vi "IHL_Inspecting Helper.vi"(8 "error in (no error)":errorcluster, 10 "Inspect Helper Loop Data":T2={"IHL State"=enum."Init", "Timeout"=0, "Loop Count"=0, "Start Sample No."=0, "No. Samples"=0, "Collecting Data"=FALSE, "Success Flag"=FALSE, "Inspect Status "={"Ready"=FALSE, "Inspecting"=FALSE, "Cancel"=FALSE}, "Status"=0, "Encoder Count"=0, "PosToStartScan"=50800, "ScanLength"=50800, "MaxSamples"=50800, "PosToEndScan"=0, "data value reference"=refnum, "Block Cnt notifier out"=refnum, "EventLog"=refnum}) -> (0 "error out":errorcluster, 2 "Inspect Helper Loop Data out":T2={"IHL State"=enum."Init", "Timeout"=0, "Loop Count"=0, "Start Sample No."=0, "No. Samples"=0, "Collecting Data"=FALSE, "Success Flag"=FALSE, "Inspect Status "={"Ready"=FALSE, "Inspecting"=FALSE, "Cancel"=FALSE}, "Status"=0, "Encoder Count"=0, "PosToStartScan"=50800, "ScanLength"=50800, "MaxSamples"=50800, "PosToEndScan"=0, "data value reference"=refnum, "Block Cnt notifier out"=refnum, "EventLog"=refnum}, 3 "State String":string="IHL:Timeout: Inspecting")   [LabVIEW 2015, in "Tool Module.lvlib"]
uses:
  Tool Module.lvlib
  _IHL Data Cluster--typedef.ctl
  Event Logger Library/Event Log/EventLog.lvclass
  _IHL SM Enum--typedef.ctl
  _IHL Status Update Cluster--typedef.ctl
  _Sample Data Rtn Cluster--typedef.ctl
  _Inspection Limits cluster--typedef.ctl
panel:
  out "latest notification":T1
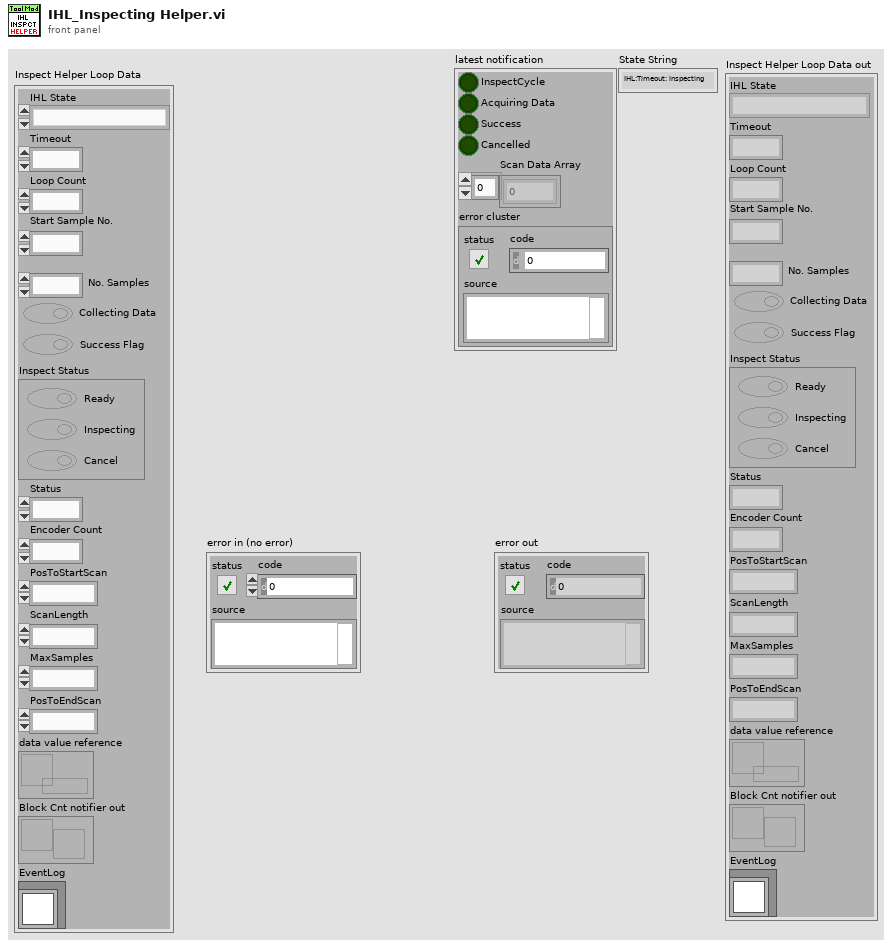
[diagram p1: front panel]
types:
  T1 = typedef "Tool Module.lvlib/_Sample Data Rtn Cluster--typedef.ctl" = cluster{"InspectCycle":bool, "Acquiring Data":bool, "Success":bool, "Cancelled":bool, "Scan Data Array":u32[], "error cluster":errorcluster}
  T2 = typedef "Tool Module.lvlib/_IHL Data Cluster--typedef.ctl" = cluster{"IHL State":T3, "Timeout":i32, "Loop Count":i32, "Start Sample No.":u32, "No. Samples":i32, "Collecting Data":bool, "Success Flag":bool, "Inspect Status ":T4, "Status":u16, "Encoder Count":i32, "PosToStartScan":i32, "ScanLength":i32, "MaxSamples":i32, "PosToEndScan":i32, "data value reference":refnum<data-value>, "Block Cnt notifier out":refnum<notifier>, "EventLog":refnum<class "EventLog.lvclass">}
  T3 = typedef "Tool Module.lvlib/_IHL SM Enum--typedef.ctl" = enum16{"Init", "Set Motion Speed", "Move To Scan Start", "Wait for Motion Out", "Wait for Start Pos", "Inspect: START", "Wait for Motion IN", "Wait for Inspect Range", "Inspecting", "Inspect: STOP"}
  T4 = typedef "Tool Module.lvlib/_IHL Status Update Cluster--typedef.ctl" = cluster{"Ready":bool, "Inspecting":bool, "Cancel":bool}
  T5 = typedef "Tool Module.lvlib/_Inspection Limits cluster--typedef.ctl" = cluster{"MaxSamples":i32, "PosToStartScan":i32, "PosToEndScan":i32, "ScanLength":i32}
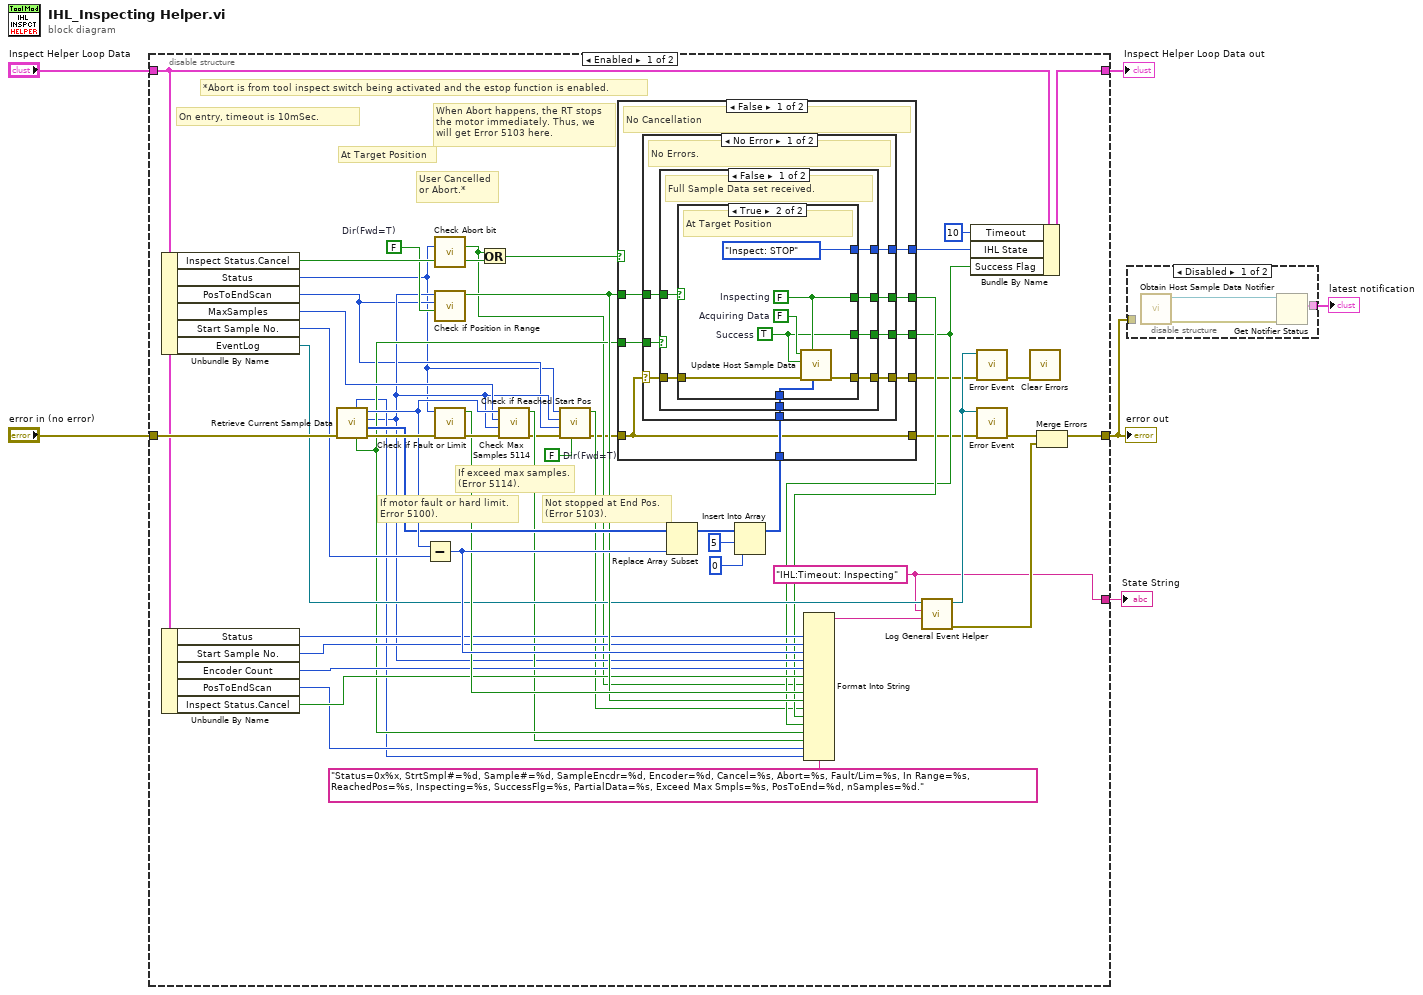
[diagram p0: block diagram]
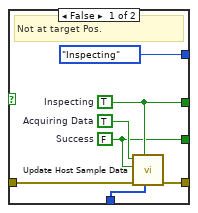
[diagram p3: hidden frame]
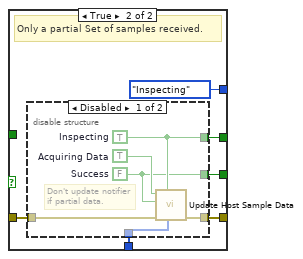
[diagram p4: hidden frame]
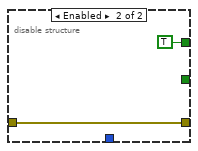
[diagram p5: hidden frame]
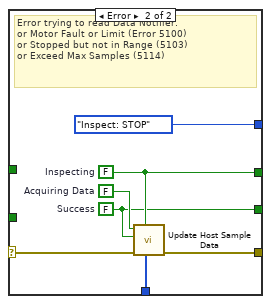
[diagram p6: hidden frame]
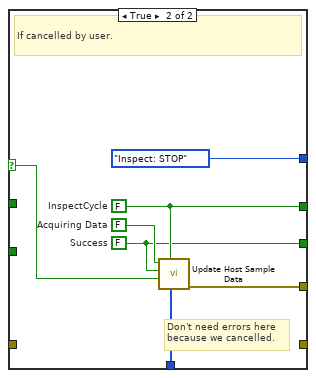
[diagram p7: hidden frame]
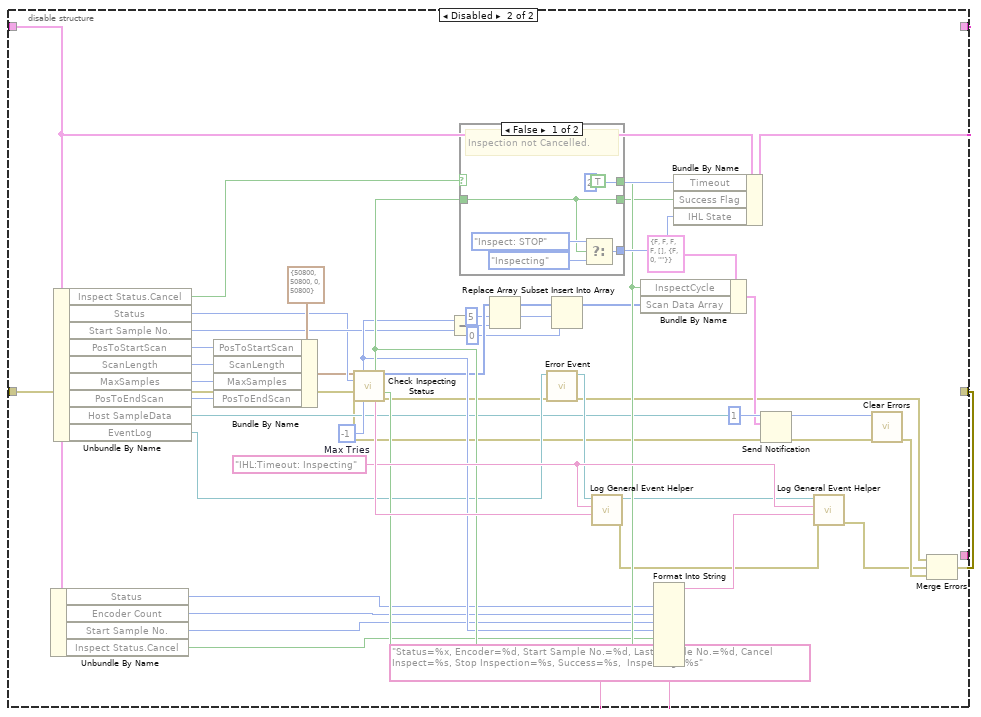
[diagram p8: hidden frame]
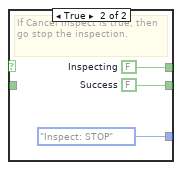
[diagram p9: hidden frame]
diagram:
  n1 = disable-structure shown="Enabled" {
    disable-tunnel: "Inspect Helper Loop Data" -> [w29 w125]
    disable-tunnel: [w30 w124] -> w5
    disable-tunnel: [w28 w123] -> w1
    disable-tunnel: "error in (no error)" -> [w55 w122]
    disable-tunnel: [w9 _] -> w2
    frame Enabled {
      w22 = FALSE  # Dir(Fwd=T)
      w9 = "IHL:Timeout: Inspecting"
      w53 = FALSE  # Dir(Fwd=T)
      # "When Abort happens, the RT stops the motor immediately. Thus, we will get Error 5103 here."
      # "On entry, timeout is 10mSec."
      # "Not stopped at End Pos.\n(Error 5103)."
      # "*Abort is from tool inspect switch being activated and the estop function is enabled."
      # "User Cancelled\nor Abort.*"
      # "At Target Position"
      # "If motor fault or hard limit.\nError 5100)."
      # "If exceed max samples.\n(Error 5114)."
      n2 = Unbundle By Name(w29) -> ("Inspect Status.Cancel"=w56:bool, "Status"=w19:u16, "PosToEndScan"=w20:i32, "MaxSamples"=w34:i32, "Start Sample No."=w41:u32, "EventLog"=w33:refnum<class "EventLog.lvclass">)
      n3 = Unbundle By Name(w29) -> ("Status"=w37:u16, "Start Sample No."=w36:u32, "Encoder Count"=w35:i32, "PosToEndScan"=w25:i32, "Inspect Status.Cancel"=w38:bool)
      n4 = call "Retrieve Current Sample Data.vi"("error in (no error)"=w55) -> ("error out"=w54:errorcluster, "Last Sample"=w46:u32[], "Encoder Out"=w21:i32, "Last Sample No."=w51:u32, "Partial Data"=w27:bool, "nSamples"=w24:u32)  [unwired: 5 in]
      n5 = Subtract(x=w51, y=w41) -> (x-y=w42:u32)
      n6 = call "Check Abort bit.vi"("Status Byte"=w19) -> ("Abort?"=w10:bool)  [unwired: 14 in]
      n7 = call "Check if Position in Range.vi"("Dir(Fwd=T)"=w53, "Target Position"=w20, "Cur Encoder Value"=w21) -> ("In Range?"=w39:bool)  [unwired: 7 in, 1 out]
      n8 = call "Check if Fault or Limit.vi"("error in (no error)"=w54, "Status In"=w19) -> ("error out"=w52:errorcluster, "Fault or Limit"=w40:bool)  [unwired: 8 in]
      n9 = Or(x=w10, y=w56) -> (x .or. y?=w16:bool)
      n10 = call "Check Max Samples 5114.vi"("error in (no error)"=w52, "Encoder"=w21, "Max Samples"=w34, "Sample Count"=w51) -> ("error out"=w23:errorcluster, "Exceed Max?"=w26:bool)  [unwired: 6 in]
      n11 = call "Check if Reached Start Pos.vi"("Dir(Fwd=T)"=w22, "error in (no error)"=w23, "Target Encdr Pos."=w20, "Cur Encoder Value"=w21, "Status Byte"=w19) -> ("error out"=w8:errorcluster, "ReachedPos?"=w13:bool)  [unwired: 2 in, 3 out]
      n12 = Replace Array Subset(array=w46, new element=w42) -> (w49:u32[])  [unwired: 1 in]
      n13 = Insert Into Array(array=w49, index=5, new element=u32 0 ("new element/subarray")) -> (w11:u32[])
      n14 = case shown="False" w16 {
        selector: w16 -> [_ w115]
        tunnel: w39 -> [w64 _]
        tunnel: [w63 _IHL_SM_Enum--typedef."Inspect: STOP" ("Inspect State")] -> w50
        tunnel: [w62 w116] -> w17
        tunnel: [w61 w118] -> w18
        tunnel: w27 -> [w60 _]
        tunnel: [w59 w120] -> w12
        tunnel: w11 -> [w58 w119]
        tunnel: w8 -> [w57 _]
        tunnel: [w57 _] -> w7
        frame False {
          # "No Cancellation"
          n15 = case shown="No Error" w57 {
            selector: w57 -> [w67 w108]
            tunnel: w64 -> [w72 _]
            tunnel: [w71 _IHL_SM_Enum--typedef."Inspect: STOP" ("Inspect State")] -> w63
            tunnel: [w70 w109] -> w62
            tunnel: [w69 w111] -> w61
            tunnel: w60 -> [w68 _]
            tunnel: [w66 w113] -> w59
            tunnel: w58 -> [w65 w112]
            frame No Error {
              # "No Errors."
              n16 = case shown="False" w68 {
                tunnel: w72 -> [w79 _]
                tunnel: [w78 _IHL_SM_Enum--typedef."Inspecting" ("Inspect State")] -> w71
                tunnel: [w77 w94] -> w70
                tunnel: [w76 w95] -> w69
                tunnel: w67 -> [w75 w97]
                tunnel: [w74 w98] -> w66
                tunnel: w65 -> [w73 w96]
                frame False {
                  # "Full Sample Data set received."
                  n17 = case shown="True" w79 {
                    tunnel: [_IHL_SM_Enum--typedef."Inspecting" ("Inspect State") _IHL_SM_Enum--typedef."Inspect: STOP" ("Inspect State")] -> w78
                    tunnel: [w82 w90] -> w77
                    tunnel: [w84 w92] -> w76
                    tunnel: w75 -> [w80 w89]
                    tunnel: [w85 w88] -> w74
                    tunnel: w73 -> [w81 w87]
                    frame False {
                      w82 = FALSE  # Success
                      w83 = TRUE  # Acquiring Data
                      w84 = TRUE  # Inspecting
                      # "Not at target Pos."
                      n18 = call "Update Host Sample Data.vi"("Scan Data Array"=w81, "InspectCycle"=w84, "error in (no error)"=w80, "Success"=w82, "Acquiring Data"=w83) -> ("error out"=w85:errorcluster)  [unwired: 6 in]
                    }
                    frame True {
                      w91 = FALSE  # Acquiring Data
                      w92 = FALSE  # Inspecting
                      w90 = TRUE  # Success
                      # "At Target Position"
                      n19 = call "Update Host Sample Data.vi"("Scan Data Array"=w87, "InspectCycle"=w92, "error in (no error)"=w89, "Success"=w90, "Acquiring Data"=w91) -> ("error out"=w88:errorcluster)  [unwired: 6 in]
                    }
                  }
                }
                frame True {
                  # "Only a partial Set of samples received."
                  n20 = disable-structure shown="Disabled" {
                    disable-tunnel: [w105 w107] -> w98
                    disable-tunnel: w97 -> [w104 w107]
                    disable-tunnel: w96 -> [w103 _]
                    disable-tunnel: [w102 TRUE ("Inspecting")] -> w95
                    disable-tunnel: [w100 _] -> w94
                    frame Disabled {
                      w102 = TRUE  # Inspecting
                      w101 = TRUE  # Acquiring Data
                      w100 = FALSE  # Success
                      # "Don't update notifier if partial data."
                      n21 = call "Update Host Sample Data.vi"("Scan Data Array"=w103, "InspectCycle"=w102, "error in (no error)"=w104, "Success"=w100, "Acquiring Data"=w101) -> ("error out"=w105:errorcluster)  [unwired: 6 in]
                    }
                    frame Enabled {
                    }
                  }
                }
              }
            }
            frame Error {
              w109 = FALSE  # Success
              w110 = FALSE  # Acquiring Data
              w111 = FALSE  # Inspecting
              # "Error trying to read Data Notifier.\nor Motor Fault or Limit (Error 5100)\nor Stopped but not in Range (5103)\nor Exceed Max Samples (5114)"
              n22 = call "Update Host Sample Data.vi"("Scan Data Array"=w112, "InspectCycle"=w111, "error in (no error)"=w108, "Success"=w109, "Acquiring Data"=w110) -> ("error out"=w113:errorcluster)  [unwired: 6 in]
            }
          }
        }
        frame True {
          w116 = FALSE  # Success
          w118 = FALSE  # InspectCycle
          w117 = FALSE  # Acquiring Data
          # "Don't need errors here because we cancelled."
          # "If cancelled by user."
          n23 = call "Update Host Sample Data.vi"("Scan Data Array"=w119, "InspectCycle"=w118, "Cancelled"=w115, "Success"=w116, "Acquiring Data"=w117) -> ("error out"=w120:errorcluster)  [unwired: 6 in]
        }
      }
      n24 = Format Into String(format string="Status=0x%x, StrtSmpl#=%d, Sample#=%d, SampleEncdr=%d, Encoder=%d, Cancel=%s, Abort=%s, Fault/Lim=%s, In Range=%s, ReachedPos=%s, Inspecting=%s, SuccessFlg=%s, PartialData=%s, Exceed Max Smpls=%s, PosToEnd=%d, nSamples=%d.", w37, w36, w42, w21, w35, w38, w10, w40, w39, w13, w18, w17, w27, w26, w25, w24) -> (resulting string=w32:string)  [unwired: 2 in, 1 out]
      n25 = call "Log General Event Helper.vi"("Payload"=w32, "State Info"=w9, "EventLog in"=w33) -> ("error out"=w31:errorcluster, "EventLog out"=w15:refnum<class "EventLog.lvclass">)  [unwired: 7 in]
      n26 = Bundle By Name(cluster=w29, "Timeout"=10, "IHL State"=w50, "Success Flag"=w17) -> (w30:T2)
      n27 = call "Error Event.vi"("error in (no error)"=w12, "EventLog ref"=w15) -> ("error out"=w14:errorcluster)  [unwired: 8 in, 1 out]
      n28 = call "Error Event.vi"("error in (no error)"=w7, "EventLog ref"=w15) -> ("error out"=w44:errorcluster)  [unwired: 8 in, 1 out]
      n29 = call <vilib>:"Clear Errors.vi"("error in (no error)"=w14) -> ()  [unwired: 5 in, 2 out]
      n30 = Merge Errors(w44, w31) -> (w28:errorcluster)
    }
    frame Disabled {
      w138 = -1  # Max Tries
      w166 = "IHL:Timeout: Inspecting"
      n31 = Unbundle By Name(w125) -> ("Status"=w154:u16, "Encoder Count"=w155:i32, "Start Sample No."=w156:u32, "Inspect Status.Cancel"=w158:bool)
      n32 = Unbundle By Name(w125) -> ("Inspect Status.Cancel"=w149:bool, "Status"=w137:u16, "Start Sample No."=w140:u32, "PosToStartScan"=w133:i32, "ScanLength"=w134:i32, "MaxSamples"=w135:i32, "PosToEndScan"=w136:i32, "Host SampleData"=w128:refnum<notifier>, "EventLog"=w130:refnum<class "EventLog.lvclass">)
      n33 = Bundle By Name(cluster=T5 {"MaxSamples"=50800, "PosToStartScan"=50800, "PosToEndScan"=0, "ScanLength"=50800} ("Inspection Limits"), "PosToStartScan"=w133, "ScanLength"=w134, "MaxSamples"=w135, "PosToEndScan"=w136) -> (w132:T5)
      n34 = call "Check Inspecting Status.vi"("Inspection Limits"=w132, "Status Byte"=w137, "Max Tries"=w138) -> ("Last Sample No."=w157:u32, "Stop Inspection"=w159:bool, "Last Sample"=w145:u32[], "Success"=w161:bool, "DebugLog String"=w167:string, "error out"=w129:errorcluster)  [unwired: 5 in, 2 out]
      n35 = Subtract(x=w157, y=w140) -> (x-y=w144:u32)
      n36 = case shown="False" w149 {
        tunnel: w159 -> [w170 _]
        tunnel: [TRUE w175] -> w160
        tunnel: [w172 _IHL_SM_Enum--typedef."Inspect: STOP" ("Inspect State")] -> w169
        tunnel: [w170 w176] -> w147
        frame False {
          # "Inspection not Cancelled."
          n37 = Select(t=_IHL_SM_Enum--typedef."Inspect: STOP" ("Inspect State"), s=w170, f=_IHL_SM_Enum--typedef."Inspecting" ("Inspect State")) -> (s? t:f=w172:T3)
        }
        frame True {
          w175 = FALSE  # Inspecting
          w176 = FALSE  # Success
          # "If Cancel Inspect is true, then go stop the inspection."
        }
      }
      n38 = Replace Array Subset(array=w145, new element=w144) -> (w143:u32[])  [unwired: 1 in]
      n39 = call "Error Event.vi"("error in (no error)"=w129, "EventLog ref"=w130) -> ("error out"=w139:errorcluster, "EventLog ref"=w165:refnum<class "EventLog.lvclass">)  [unwired: 8 in]
      n40 = Insert Into Array(array=w143, index=5, new element=u32 0 ("new element/subarray")) -> (w148:u32[])
      n41 = call "Log General Event Helper.vi"("Payload"=w167, "State Info"=w166, "EventLog in"=w165) -> ("error out"=w126:errorcluster, "EventLog out"=w127:refnum<class "EventLog.lvclass">)  [unwired: 7 in]
      n42 = Bundle By Name(cluster=T1 {"InspectCycle"=FALSE, "Acquiring Data"=FALSE, "Success"=FALSE, "Cancelled"=FALSE, "Scan Data Array"=[], "error cluster"={"status"=FALSE, "code"=0, "source"=""}} ("_Full Scan Data Rtn Cluster"), "InspectCycle"=w160, "Scan Data Array"=w148) -> (w150:T1)
      n43 = Format Into String(format string="Status=%x, Encoder=%d, Start Sample No.=%d, Last Sample No.=%d, Cancel Inspect=%s, Stop Inspection=%s, Success=%s,  Inspecting=%s", w154, w155, w156, w157, w158, w159, w161, w160) -> (resulting string=w153:string)  [unwired: 2 in, 1 out]
      n44 = Bundle By Name(cluster=w125, "Timeout"=2, "Success Flag"=w147, "IHL State"=w169) -> (w124:T2)
      n45 = Send Notification(notification=w150, notifier=w128, error in (no error)=w122) -> (error out=w151:errorcluster)  [unwired: 1 out]
      n46 = call "Log General Event Helper.vi"("error in (no error)"=w126, "Payload"=w153, "State Info"=w166, "EventLog in"=w127) -> ("error out"=w131:errorcluster)  [unwired: 6 in, 1 out]
      n47 = call <vilib>:"Clear Errors.vi"("error in (no error)"=w151, "specific error code to clear (0: all)"=1) -> ("error out"=w163:errorcluster)  [unwired: 4 in, 1 out]
      n48 = Merge Errors(w139, w131, w163) -> (w123:errorcluster)
    }
  }
  "error out" <- w1
  "Inspect Helper Loop Data out" <- w5
  "State String" <- w2
  n49 = disable-structure shown="Disabled" {
    disable-tunnel: [w180 _] -> w3
    disable-tunnel: w1 -> [_ _]
    frame Disabled {
      n50 = call "Obtain Host Sample Data Notifier.vi"() -> ("error out"=w179:errorcluster, "Sample Data Notifier"=w178:refnum<notifier>)  [unwired: 10 in]
      n51 = Get Notifier Status(notifier=w178, error in (no error)=w179) -> (current notification=w180:T1)  [unwired: 4 out]
    }
    frame Enabled {
    }
  }
  "latest notification" <- w3
